vi "batteryCheckerPlayground.vi"() -> ()   [LabVIEW 2017]
uses:
  Sensors/Power Sensor - Adafruit INA219/INA219 Measurements.ctl
panel:
  in  "Reset":bool
  in  "Iteration Skip":i32=10
  out "Total Capacity":dbl format="%.1f W-s"
  out "Power Used":dbl format="%.1f W-s"
  out "Battery Charge":dbl(slide) scale=0.0..100.0
  in  "Simulated Power Use (W)":dbl(slide) scale=0.0..1000.0
  out "Battery Power Reading":T1 {"Current" format="%#.3g A"; "Power" format="%#.3g W"; "Shunt Voltage" format=" %#.3g V"; "Bus Voltage" format="%#.3g V"; "Voltage (Total)" format="%#.3g V"}
  out "Error Out":errorcluster
  in  "Error In":errorcluster
  in  "Stop SImulation VI":bool
  # "Directions for simulator:\n1. Run the VI\n2. Adjust the Simulated Power Use (W) to see impact on power consumption\n3. Once battery is recharged, hit Reset button to see Power Used reset to 0 and Battery Charge to 100%\n4. If writing to file is causing issues with code performance, adjust Iteration Skip. This skips N power readings before writing to file.\n5. Stop VI and rerun to see the Battery Charge pick up where it left off. Try power cycling as well.\n6. Hit Stop SImulation VI to end simulation\n\nNOTE: Please double check my math in the batteryMonitor subVI in the monitor state."
  # "Note: Ignoring all data but Power and Time Stamp"
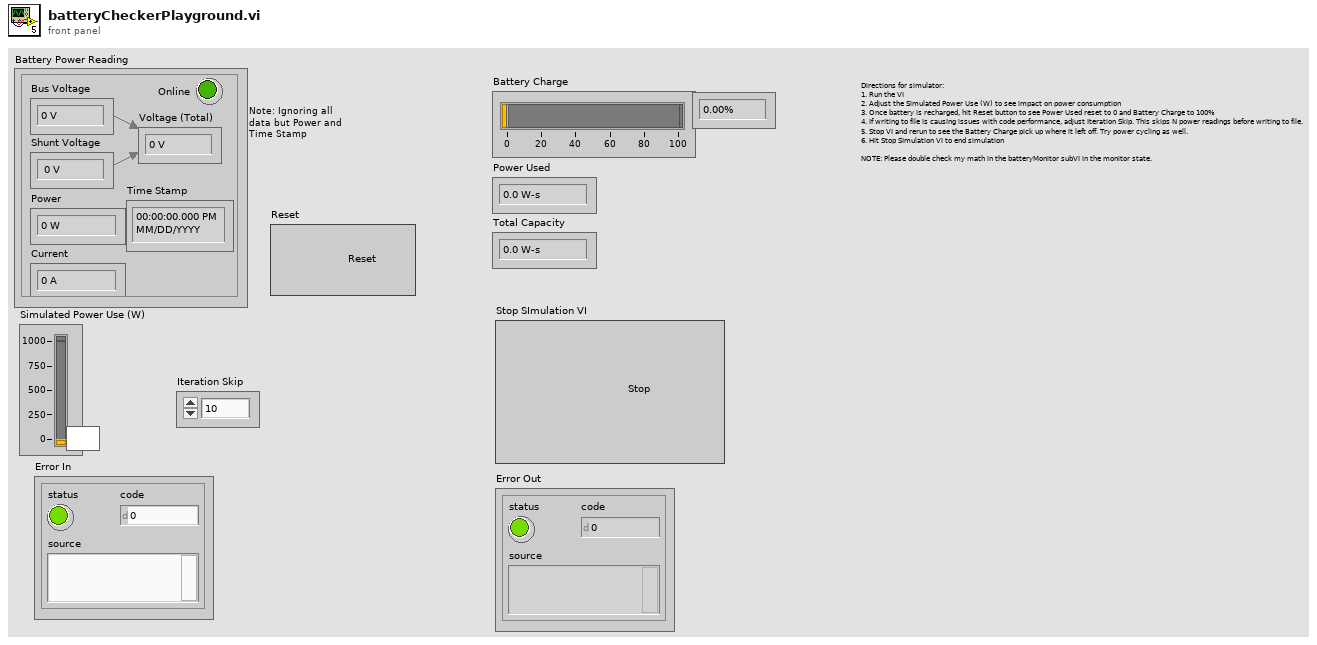
[diagram p1: front panel]
types:
  T1 = typedef "INA219 Measurements.ctl" = cluster{"Voltage (Total)":dbl, "Bus Voltage":dbl, "Shunt Voltage":dbl, "Power":dbl, "Current":dbl, "Online":bool, "Time Stamp":timestamp}
  T2 = enum16{"Monitor", "Initialize", "Reset", "Write to File"}
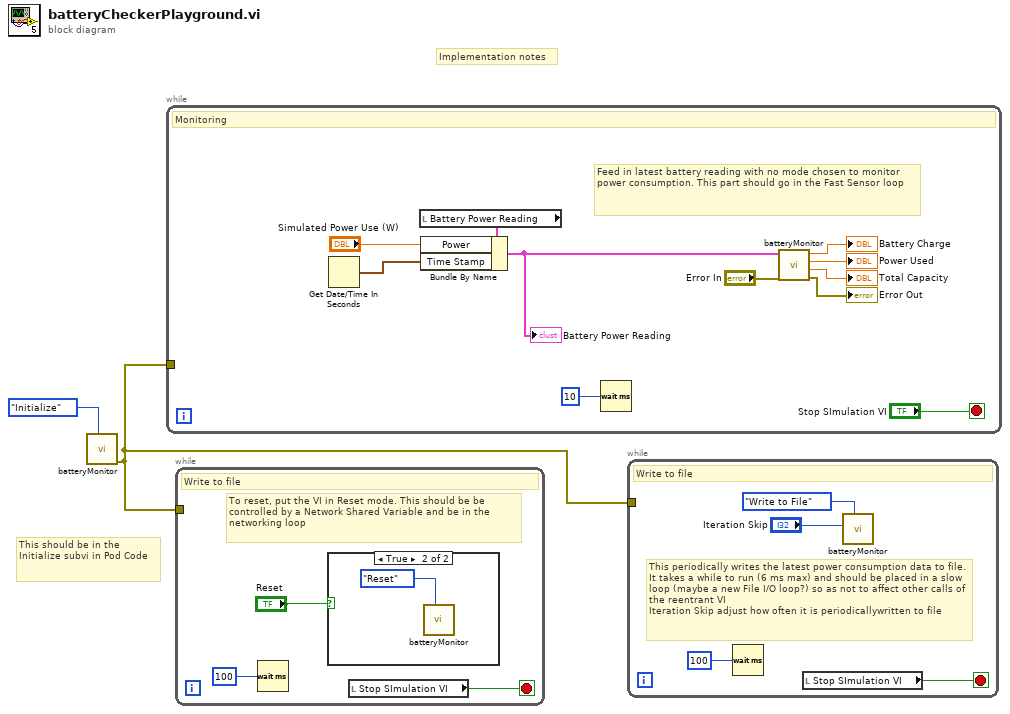
[diagram p0: block diagram]
diagram:
  # "This should be in the Initialize subvi in Pod Code"
  # "Implementation notes"
  n1 = call "batteryMonitor.vi"("Mode"=T2."Initialize") -> ("Error Out"=w1:errorcluster)  [unwired: 7 in, 3 out]
  n2 = while {
    tunnel: w1 -> [_]
    stop <- "Stop SImulation VI" stop-if-true
    # "Feed in latest battery reading with no mode chosen to monitor power consumption. This part should go in the Fast Sensor loop"
    # "Monitoring"
    n3 = Get Date/Time In Seconds() -> (seconds since 1Jan1904=w10:timestamp)
    n4 = local read "Battery Power Reading"() -> (w12:T1)
    n5 = Bundle By Name(cluster=w12, "Power"="Simulated Power Use (W)", "Time Stamp"=w10) -> (w9:T1)
    "Battery Power Reading" <- w9
    n6 = Wait (ms)(milliseconds to wait=u32 10 ("millisecond timer value")) -> ()  [unwired: 1 out]
    n7 = call "batteryMonitor.vi"("Error In"="Error In", "Battery Power Reading"=w9) -> ("Error Out"=→"Error Out":errorcluster, "Total Capacity"=→"Total Capacity":dbl, "Power Used"=→"Power Used":dbl, "Battery Charge"=→"Battery Charge":dbl)  [unwired: 6 in]
  }
  n8 = while {
    tunnel: w1 -> [_]
    stop <- w16 stop-if-true
    # "To reset, put the VI in Reset mode. This should be be controlled by a Network Shared Variable and be in the networking loop"
    # "Write to file"
    n9 = Wait (ms)(milliseconds to wait=u32 100 ("millisecond timer value")) -> ()  [unwired: 1 out]
    n10 = case shown="True" "Reset" {
      frame False {
      }
      frame True {
        n11 = call "batteryMonitor.vi"("Mode"=T2."Reset") -> ()  [unwired: 7 in, 4 out]
      }
    }
    n12 = local read "Stop SImulation VI"() -> (w16:bool)
  }
  n13 = while {
    tunnel: w1 -> [_]
    stop <- w21 stop-if-true
    # "This periodically writes the latest power consumption data to file. It takes a while to run (6 ms max) and should be placed in a slow loop (maybe a new File I/O loop?) so as not to affect other calls of the reentrant VI\nIteration Skip adjust how often it is periodicallywritten to file"
    # "Write to file"
    n14 = Wait (ms)(milliseconds to wait=u32 100 ("millisecond timer value")) -> ()  [unwired: 1 out]
    n15 = local read "Stop SImulation VI"() -> (w21:bool)
    n16 = call "batteryMonitor.vi"("Mode"=T2."Write to File", "Iteration Skip"="Iteration Skip") -> ()  [unwired: 6 in, 4 out]
  }
